vi "Read Sampling Interval.vi"(8 "error in (no error)":errorcluster, 11 "OD600 in":refnum<class "OD600.lvclass">) -> (0 "error out":errorcluster, 2 "Sampling Interval":refnum<vi>, 3 "OD600 out":refnum<class "OD600.lvclass">)   [LabVIEW 2013, in "OD600.lvlib" / "OD600.lvclass"]
uses:
  OD600.lvclass
  OD600.lvclass/OD600.ctl
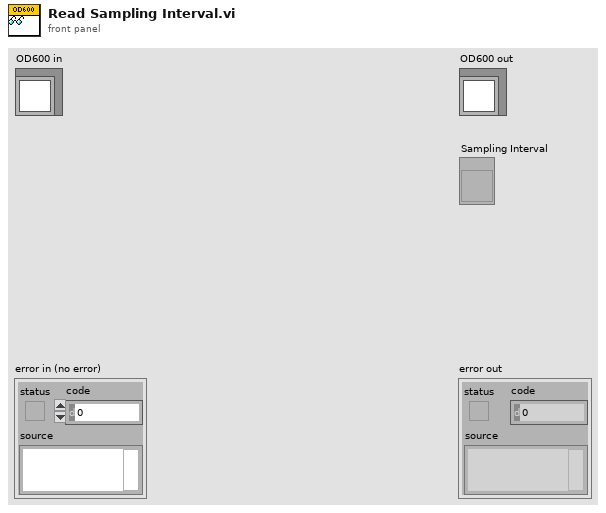
[diagram p1: front panel]
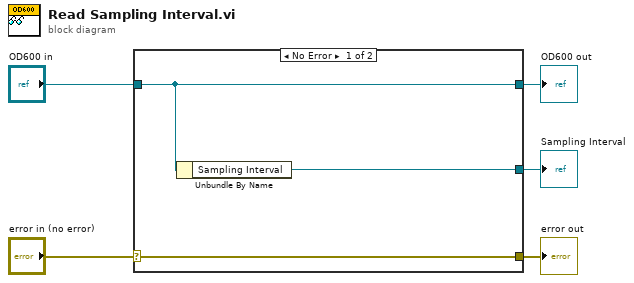
[diagram p0: block diagram]
diagram:
  n1 = case shown="No Error" "error in (no error)" {
    selector: "error in (no error)" -> [w8 w9]
    tunnel: [w8 w9] -> w4
    tunnel: [w7 w10] -> w2
    tunnel: "OD600 in" -> [w7 w10]
    tunnel: [w6 _] -> w1
    frame No Error {
      n2 = Unbundle By Name(w7) -> ("Sampling Interval"=w6:refnum<vi>)
    }
    frame Error {
    }
  }
  "error out" <- w4
  "OD600 out" <- w2
  "Sampling Interval" <- w1
